vi "TCPRouter ClientAPI Example 1.2.vi"() -> ()   [LabVIEW 2020]
uses:
  01bf6535-069d-4827-9114-7ea8e28c608a.vi
  <userlib>/_NEVSTOP/Communicable State Machine(CSM)/addons/MassData-Parameter/_support/FGV-MassData.vi
  _addons/TCP-Router/ClientAPI/TcpRouter-Client.lvclass
panel:
  out "Waveform Graph":dbl[](graph)
  out "wait(ms)":u32
  out "Server Ready?":bool
  out "Response":string="DoA"
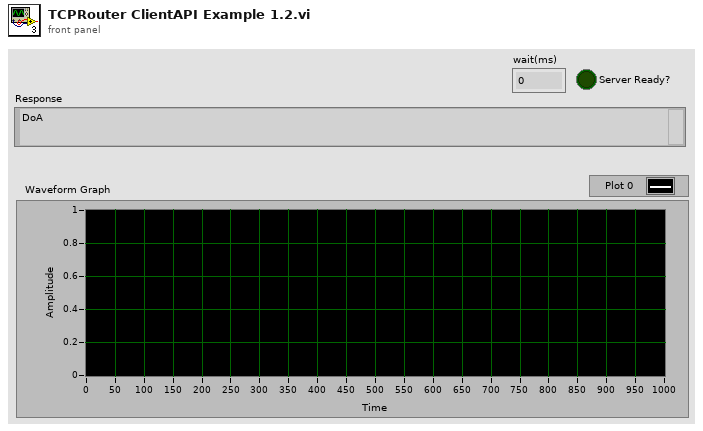
[diagram p1: front panel]
types:
  T1 = cluster{"IP Address":string, "Port":u16, "ConnectTMO":i32}
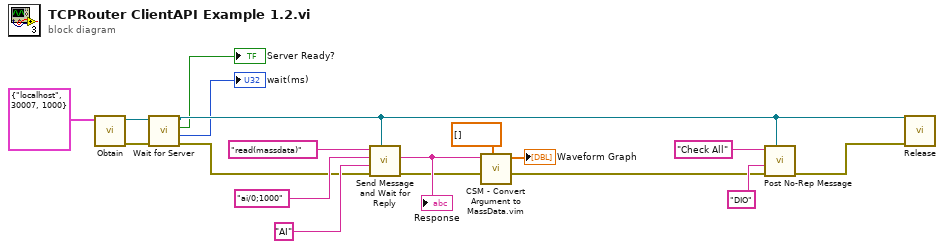
[diagram p0: block diagram]
diagram:
  n1 = call "Obtain.vi"("Connection"=T1 {"IP Address"="localhost", "Port"=30007, "ConnectTMO"=1000}) -> ("error out"=w11:errorcluster, "TcpRouter-Client out"=w10:refnum<class "TcpRouter-Client.lvclass">)  [unwired: 9 in]
  n2 = call "Wait for Server.vi"("error in (no error)"=w11, "TcpRouter-Client in"=w10) -> ("error out"=w9:errorcluster, "wait(ms)"=→"wait(ms)":u32, "Server Ready?"=→"Server Ready?":bool, "TcpRouter-Client out"=w8:refnum<class "TcpRouter-Client.lvclass">)  [unwired: 6 in]
  n3 = call "Send Message and Wait for Reply.vi"("TcpRouter-Client in"=w8, "error in (no error)"=w9, "Target Module"="AI", "Arguments (\"\")"="ai/0;1000" ("State"), "State"="read(massdata)") -> ("error out"=w4:errorcluster, "Response"=w7:string)  [unwired: 5 in]
  "Response" <- w7
  n4 = call "CSM - Convert Argument to MassData.vim"("Type"=dbl[] [], "error in (no error)"=w4, "MassData Argument"=w7) -> ("error out"=w3:errorcluster, "Data"=→"Waveform Graph":dbl[])  [unwired: 5 in]
  n5 = call "Post No-Rep Message.vi"("TcpRouter-Client in"=w8, "error in (no error)"=w3, "Target Module"="DIO", "State"="Check All") -> ("error out"=w14:errorcluster)  [unwired: 7 in]
  n6 = call "Release.vi"("error in (no error)"=w14, "TcpRouter-Client in"=w8) -> ()  [unwired: 9 in, 1 out]
